vi "To Variant Attributes.vi"(8 "error in (no error)":errorcluster, 11 "DapperRow in":refnum<class "DapperRow.lvclass">) -> (0 "error out":errorcluster, 2 "DbRow":variant, 3 "DapperRow out":refnum<class "DapperRow.lvclass">)   [LabVIEW 2020, in "ORM_Dapper.lvlib" / "DapperRow.lvclass"]
uses:
  DapperRow.lvclass
  DapperRow.lvclass/DapperRow.ctl
  Read ref.vi
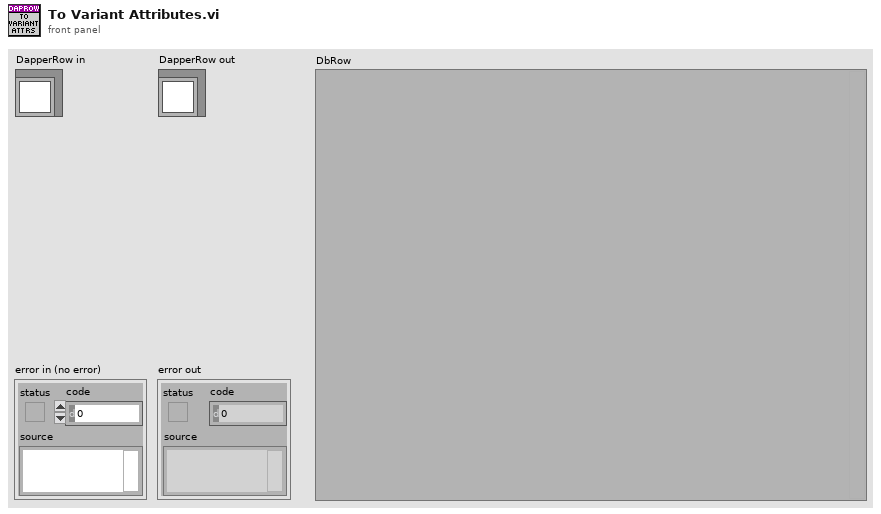
[diagram p1: front panel]
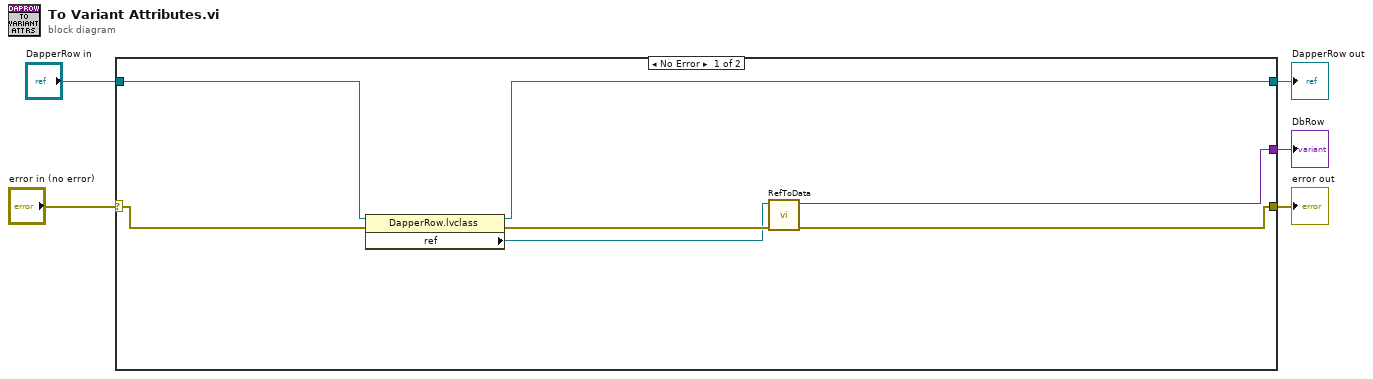
[diagram p0: block diagram]
diagram:
  n1 = case shown="No Error" "error in (no error)" {
    selector: "error in (no error)" -> [w12 w14]
    tunnel: [w10 w14] -> w4
    tunnel: [w7 w13] -> w2
    tunnel: "DapperRow in" -> [w8 w13]
    tunnel: [w11 _] -> w1
    frame No Error {
      n2 = property class="DapperRow.lvclass"(reference=w8, error in=w12) -> (reference out=w7:refnum<class "DapperRow.lvclass">, error out=w9:errorcluster, "ref"=w6:refnum<k24>)
      n3 = call "RefToData.vi"("error in (no error)"=w9, ".NET Refnum in"=w6) -> ("error out"=w10:errorcluster, "variant out"=w11:variant)  [unwired: 8 in]
    }
    frame Error {
    }
  }
  "error out" <- w4
  "DapperRow out" <- w2
  "DbRow" <- w1
